vi "Test Device Under Test_Cloneable_DQMH API.vi"() -> ()   [LabVIEW 2015]
doc: "Device Under Test_Cloneable_DQMH API Tester.\n____\nDelacor QMH Thermal Chamber Examples 4.0.0.21\nCopyright (c) 2018, Delacor"
uses:
  Device Under Test_Cloneable_DQMH.lvlib
panel:
  in  "Run as Singleton?":bool
  out "timed out?":bool
  in  "Update DUT Status":bool
  out "Self Test Result":bool
  out "Power State":bool
  in  "Self Test":bool
  in  "Power Off":bool
  in  "Power On":bool
  in  "Show Block Diagram":bool
  in  "Refresh Modules":bool
  out "Active Modules":string[](array[string])
  in  "Stop Module":bool
  in  "Select Module":i32(ring)=-1 caption="Select Module\nTo send Request to" items=["All"=-1]
  in  "Run New Module":bool
  in  "Hide Module Panel":bool
  in  "Show Module Panel":bool
  out "Status":string
  # "This VI tests the API for the Module."
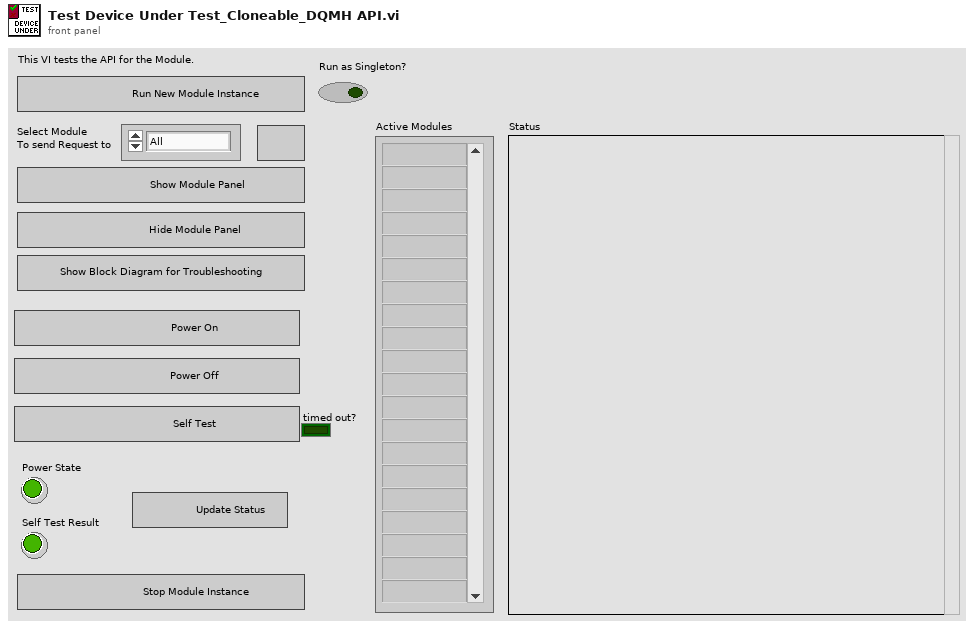
[diagram p1: front panel]
types:
  T1 = typedef "Device Under Test_Cloneable_DQMH.lvlib/Broadcast Events--cluster.ctl" = cluster{"Module Did Init":refnum<user-event>, "Status Updated":refnum<user-event>, "Error Reported":refnum<user-event>, "Module Did Stop":refnum<user-event>, "DUT Status Updated":refnum<user-event>, "Update Module Execution Status":refnum<user-event>}
  T2 = typedef "Device Under Test_Cloneable_DQMH.lvlib/Perform Self Test (Reply Payload)--cluster.ctl" = cluster{"Result":bool, "error":errorcluster}
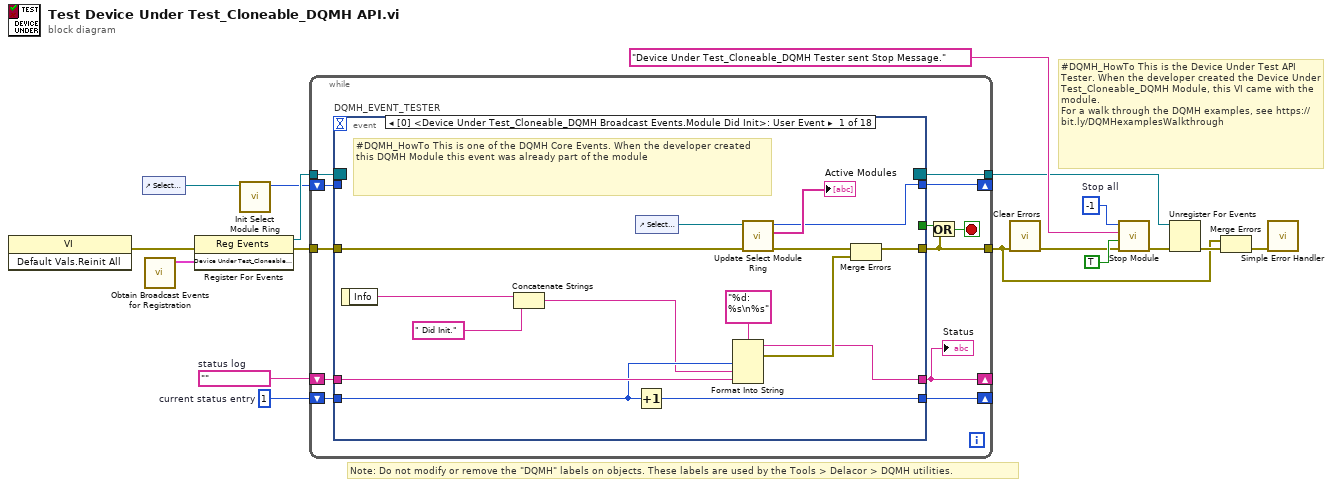
[diagram p0: block diagram]
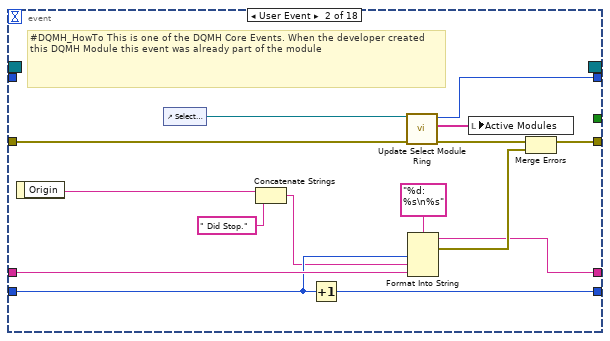
[diagram p2: hidden frame]
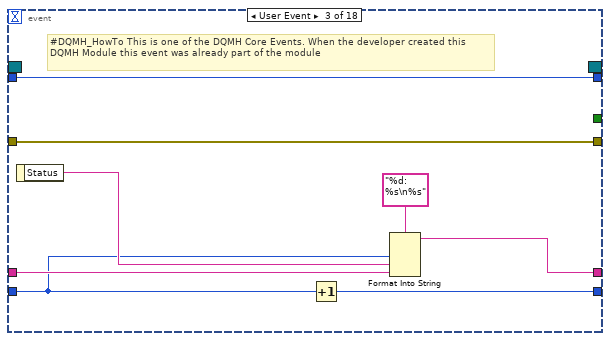
[diagram p3: hidden frame]
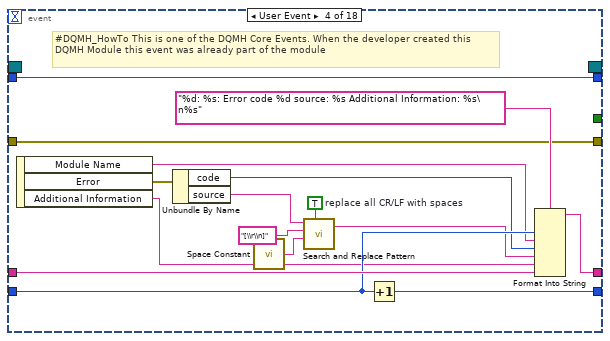
[diagram p4: hidden frame]
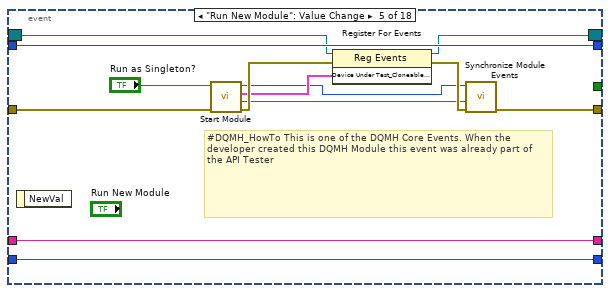
[diagram p5: hidden frame]
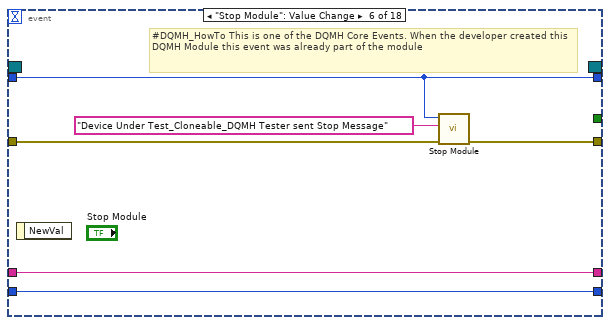
[diagram p6: hidden frame]
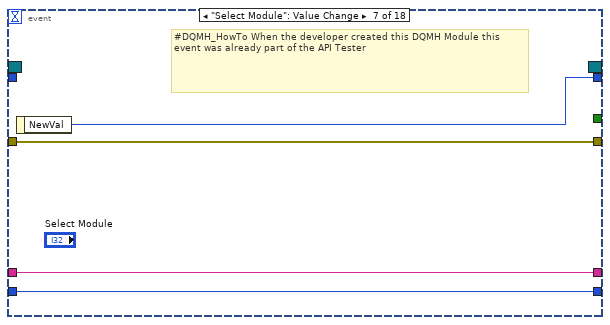
[diagram p7: hidden frame]
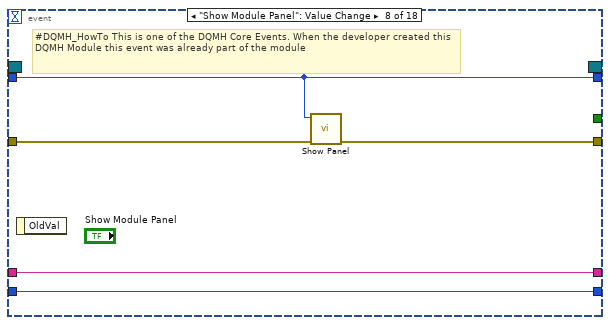
[diagram p8: hidden frame]
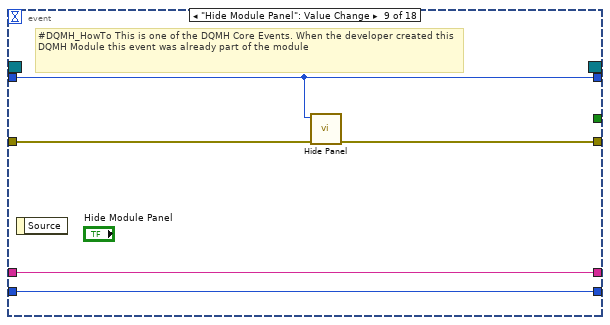
[diagram p9: hidden frame]
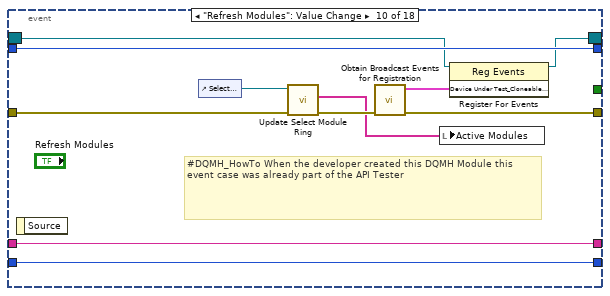
[diagram p10: hidden frame]
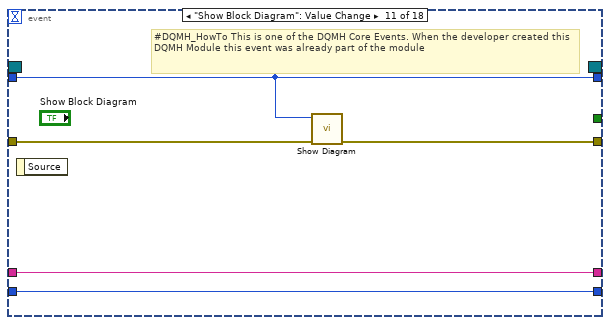
[diagram p11: hidden frame]
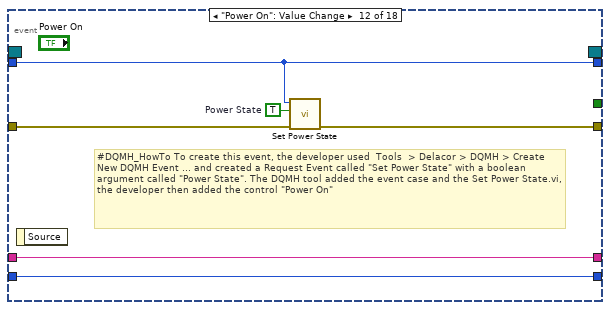
[diagram p12: hidden frame]
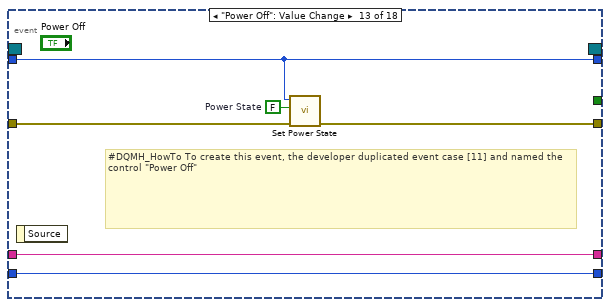
[diagram p13: hidden frame]
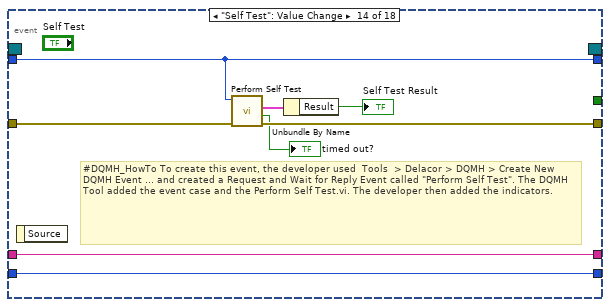
[diagram p14: hidden frame]
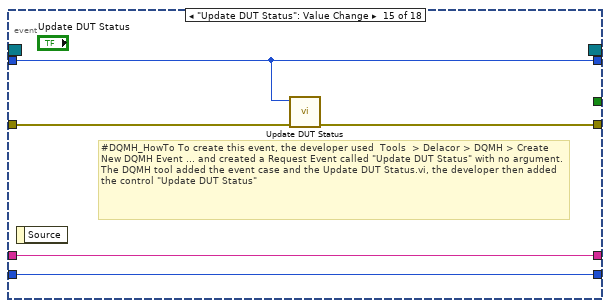
[diagram p15: hidden frame]
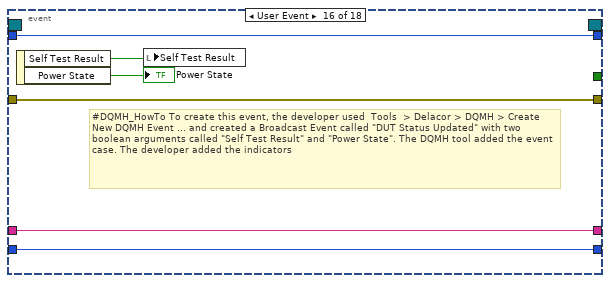
[diagram p16: hidden frame]
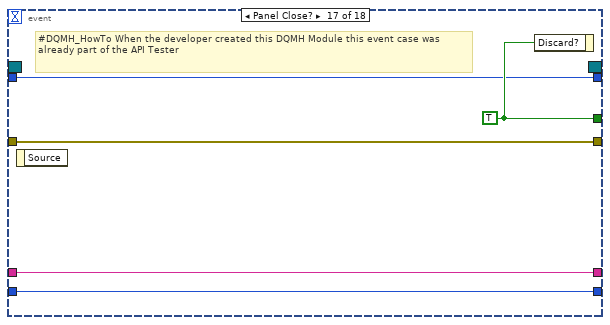
[diagram p17: hidden frame]
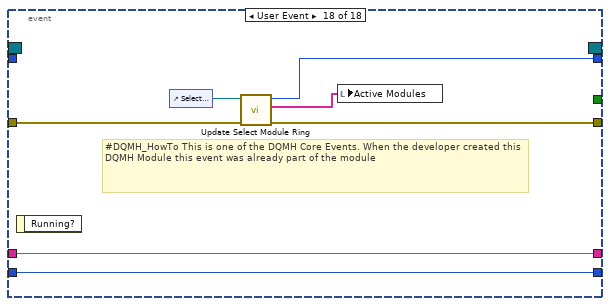
[diagram p18: hidden frame]
diagram:
  w7 = -1  # Stop all
  w13 = 1  # current status entry
  w14 = ""  # status log
  # "#DQMH_HowTo This is the Device Under Test API Tester. When the developer created the Device Under Test_Cloneable_DQMH Module, this VI came with the module.\nFor a walk through the DQMH examples, see https://bit.ly/DQMHexamplesWalkthrough"
  # "Note: Do not modify or remove the \"DQMH\" labels on objects. These labels are used by the Tools > Delacor > DQMH utilities."
  n1 = invoke class="VI" method="Default Vals.Reinit All"() -> (error out=w6:errorcluster)  [unwired: 3 in, 2 out]
  n2 = control-ref of="Select Module"() -> (w11:refnum<vi>)
  n3 = call "Obtain Broadcast Events for Registration.vi"() -> ("Device Under Test_Cloneable_DQMH Broadcast Events"=w10:T1)  [unwired: 10 in, 1 out]
  n4 = register-events(error in=w6, w10) -> (reference out=w17:refnum<event-registration>, error out=w9:errorcluster)  [unwired: 1 in]
  n5 = call "Init Select Module Ring.vi"("Select Module Ring Ref"=w11) -> ("Value for All Modules"=w12:i32)  [unwired: 8 in, 2 out]
  n6 = while {
    tunnel: w17 -> [w29]
    tunnel: [w19] -> w1
    tunnel: w9 -> [w27]
    shift-right: [w23] -> _
    shift-left: w14 -> [w25]
    shift-right: [w24] -> _
    shift-left: w13 -> [w26]
    shift-right: [w20] -> _
    shift-left: w12 -> [w21]
    tunnel: [w18] -> w5
    stop <- w22 stop-if-true
    n7 = event "DQMH_EVENT_TESTER" shown="[0] <Device Under Test_Cloneable_DQMH Broadcast Events.Module Did Init>: User Event" {
      selector: w29 -> [_ _ _ _ w90 _ _ _ _ w122 _ _ _ _ _ _ _ _]
      dyn-events: [_ _ _ _ w89 _ _ _ _ w121 _ _ _ _ _ _ _ _] -> w18
      timeout: _ -> [_ _ _ _ _ _ _ _ _ _ _ _ _ _ _ _ _ _]
      tunnel: [_ _ _ _ _ _ _ _ _ _ _ _ _ _ _ _ w168 _] -> w28
      tunnel: [w33 w51 w67 w73 w88 w98 w106 w110 w115 w118 w129 w135 w141 w149 w154 w163 w167 w172] -> w19
      tunnel: w27 -> [w35 w53 w67 w73 w91 w99 w106 w111 w116 w123 w132 w138 w144 w152 w157 w163 w167 w173]
      tunnel: w26 -> [w41 w56 w60 w79 w93 w101 w104 w108 w113 w126 w130 w136 w142 w150 w155 w161 w165 w174]
      tunnel: w25 -> [w42 w57 w63 w81 w94 w102 w105 w109 w114 w127 w131 w137 w143 w151 w156 w162 w166 w175]
      tunnel: [w39 w54 w64 w76 w94 w102 w105 w109 w114 w127 w131 w137 w143 w151 w156 w162 w166 w175] -> w23
      tunnel: [w40 w55 w66 w82 w93 w101 w104 w108 w113 w126 w130 w136 w142 w150 w155 w161 w165 w174] -> w24
      tunnel: w21 -> [_ _ w61 w83 w92 w100 _ w107 w112 w125 w128 w133 w139 w145 w153 w160 w164 _]
      tunnel: [w30 w48 w61 w83 w92 w100 w103 w107 w112 w125 w128 w133 w139 w145 w153 w160 w164 w170] -> w20
      event User Event {
        # "#DQMH_HowTo This is one of the DQMH Core Events. When the developer created this DQMH Module this event was already part of the module"
        n8 = event-data() -> ("Info"=w38:string)  [unwired: 1 in]
        n9 = Concatenate Strings(w38, " Did Init.") -> (w37:string)
        n10 = control-ref of="Select Module"() -> (w32:refnum<vi>)
        n11 = Increment(x=w41) -> (x+1=w40:i32)
        n12 = Format Into String(format string="%d: %s\n%s", w41, w37, w42) -> (resulting string=w39:string, error out=w44:errorcluster)  [unwired: 2 in]
        n13 = call "Update Select Module Ring.vi"("error in (no error)"=w35, "Select Module Ring Ref"=w32) -> ("error out"=w34:errorcluster, "Active Modules (Array)"=→"Active Modules":string[], "New Module Ring Value"=w30:i32)  [unwired: 7 in]
        n14 = Merge Errors(w34, w44) -> (w33:errorcluster)
      }
      event User Event {
        # "#DQMH_HowTo This is one of the DQMH Core Events. When the developer created this DQMH Module this event was already part of the module"
        n15 = event-data() -> ("Origin"=w46:string)  [unwired: 1 in]
        n16 = control-ref of="Select Module"() -> (w50:refnum<vi>)
        n17 = Concatenate Strings(w46, " Did Stop.") -> (w45:string)
        n18 = Increment(x=w56) -> (x+1=w55:i32)
        n19 = call "Update Select Module Ring.vi"("error in (no error)"=w53, "Select Module Ring Ref"=w50) -> ("error out"=w52:errorcluster, "Active Modules (Array)"=w49:string[], "New Module Ring Value"=w48:i32)  [unwired: 7 in]
        n20 = Format Into String(format string="%d: %s\n%s", w56, w45, w57) -> (resulting string=w54:string, error out=w59:errorcluster)  [unwired: 2 in]
        n21 = local write "Active Modules"(w49) -> ()
        n22 = Merge Errors(w52, w59) -> (w51:errorcluster)
      }
      event User Event {
        # "#DQMH_HowTo This is one of the DQMH Core Events. When the developer created this DQMH Module this event was already part of the module"
        n23 = event-data() -> ("Status"=w62:string)  [unwired: 1 in]
        n24 = Increment(x=w60) -> (x+1=w66:i32)
        n25 = Format Into String(format string="%d: %s\n%s", w60, w62, w63) -> (resulting string=w64:string)  [unwired: 2 in, 1 out]
      }
      event User Event {
        w77 = TRUE  # replace all CR/LF with spaces
        # "#DQMH_HowTo This is one of the DQMH Core Events. When the developer created this DQMH Module this event was already part of the module"
        n26 = event-data() -> ("Module Name"=w71:string, "Error"=w70:errorcluster, "Additional Information"=w68:string)  [unwired: 1 in]
        n27 = Unbundle By Name(w70) -> ("code"=w72:i32, "source"=w74:string)
        n28 = call <vilib>:"Space Constant.vi"() -> ("String"=w78:string)
        n29 = call <vilib>:"Search and Replace Pattern.vi"("string"=w74, "regular expression (\"\")"="[\\r\\n]" ("regular expression (\"\")"), "replace string (\"\")"=w78, "replace all? (F)"=w77) -> ("result string"=w75:string)  [unwired: 1 in, 1 out]
        n30 = Increment(x=w79) -> (x+1=w82:i32)
        n31 = Format Into String(format string="%d: %s: Error code %d source: %s Additional Information: %s\n%s", w79, w71, w72, w75, w68, w81) -> (resulting string=w76:string)  [unwired: 2 in, 1 out]
      }
      event "Run New Module": Value Change {
        # "#DQMH_HowTo This is one of the DQMH Core Events. When the developer created this DQMH Module this event was already part of the API Tester"
        n32 = event-data() -> ()  [unwired: 1 in, 1 out]
        n33 = call "Start Module.vi"("error in (no error)"=w91, "Run as Singleton? (F)"="Run as Singleton?") -> ("error out"=w95:errorcluster, "Wait for Event Sync?"=w87:bool, "Device Under Test_Cloneable_DQMH Broadcast Events"=w86:T1, "Module ID"=w84:i32)  [unwired: 6 in]
        n34 = register-events(reference=w90, error in=w95, w86) -> (reference out=w89:refnum<event-registration>, error out=w96:errorcluster)
        n35 = call "Synchronize Module Events.vi"("error in (no error)"=w96, "Wait for Event Sync?"=w87, "Module ID"=w84) -> ("error out"=w88:errorcluster)  [unwired: 7 in, 1 out]
      }
      event "Stop Module": Value Change {
        # "#DQMH_HowTo This is one of the DQMH Core Events. When the developer created this DQMH Module this event was already part of the module"
        n36 = event-data() -> ()  [unwired: 1 in, 1 out]
        n37 = call "Stop Module.vi"("error in (no error)"=w99, "Origin"="Device Under Test_Cloneable_DQMH Tester sent Stop Message", "Module ID"=w100) -> ("error out"=w98:errorcluster)  [unwired: 8 in]
      }
      event "Select Module": Value Change {
        # "#DQMH_HowTo When the developer created this DQMH Module this event was already part of the API Tester"
        n38 = event-data() -> ("NewVal"=w103:i32)  [unwired: 1 in]
      }
      event "Show Module Panel": Value Change {
        # "#DQMH_HowTo This is one of the DQMH Core Events. When the developer created this DQMH Module this event was already part of the module"
        n39 = event-data() -> ()  [unwired: 1 in, 1 out]
        n40 = call "Show Panel.vi"("error in (no error)"=w111, "Module ID"=w107) -> ("error out"=w110:errorcluster)  [unwired: 9 in]
      }
      event "Hide Module Panel": Value Change {
        # "#DQMH_HowTo This is one of the DQMH Core Events. When the developer created this DQMH Module this event was already part of the module"
        n41 = event-data() -> ()  [unwired: 1 in, 1 out]
        n42 = call "Hide Panel.vi"("error in (no error)"=w116, "Module ID"=w112) -> ("error out"=w115:errorcluster)  [unwired: 9 in]
      }
      event "Refresh Modules": Value Change {
        # "#DQMH_HowTo When the developer created this DQMH Module this event case was already part of the API Tester"
        n43 = event-data() -> ()  [unwired: 1 in, 1 out]
        n44 = control-ref of="Select Module"() -> (w124:refnum<vi>)
        n45 = call "Update Select Module Ring.vi"("error in (no error)"=w123, "Select Module Ring Ref"=w124) -> ("error out"=w119:errorcluster, "Active Modules (Array)"=w117:string[])  [unwired: 7 in, 1 out]
        n46 = call "Obtain Broadcast Events for Registration.vi"("error in (no error)"=w119) -> ("error out"=w118:errorcluster, "Device Under Test_Cloneable_DQMH Broadcast Events"=w120:T1)  [unwired: 9 in]
        n47 = local write "Active Modules"(w117) -> ()
        n48 = register-events(reference=w122, w120) -> (reference out=w121:refnum<event-registration>)  [unwired: 1 in, 1 out]
      }
      event "Show Block Diagram": Value Change {
        # "#DQMH_HowTo This is one of the DQMH Core Events. When the developer created this DQMH Module this event was already part of the module"
        n49 = event-data() -> ()  [unwired: 1 in, 1 out]
        n50 = call "Show Diagram.vi"("error in (no error)"=w132, "Module ID"=w128) -> ("error out"=w129:errorcluster)  [unwired: 9 in]
      }
      event "Power On": Value Change {
        w134 = TRUE  # Power State
        # "#DQMH_HowTo To create this event, the developer used  Tools  > Delacor > DQMH > Create New DQMH Event ... and created a Request Event called \"Set Power State\" with a boolean argument called \"Power State\". The DQMH tool added the event case and the Set Power State.vi, the developer then added the control \"Power On\""
        n51 = event-data() -> ()  [unwired: 1 in, 1 out]
        n52 = call "Set Power State.vi"("error in (no error)"=w138, "Power State"=w134, "Module ID"=w133) -> ("error out"=w135:errorcluster)  [unwired: 8 in]
      }
      event "Power Off": Value Change {
        w140 = FALSE  # Power State
        # "#DQMH_HowTo To create this event, the developer duplicated event case [11] and named the control \"Power Off\""
        n53 = event-data() -> ()  [unwired: 1 in, 1 out]
        n54 = call "Set Power State.vi"("error in (no error)"=w144, "Power State"=w140, "Module ID"=w139) -> ("error out"=w141:errorcluster)  [unwired: 8 in]
      }
      event "Self Test": Value Change {
        # "#DQMH_HowTo To create this event, the developer used  Tools  > Delacor > DQMH > Create New DQMH Event ... and created a Request and Wait for Reply Event called \"Perform Self Test\". The DQMH Tool added the event case and the Perform Self Test.vi. The developer then added the indicators."
        n55 = event-data() -> ()  [unwired: 1 in, 1 out]
        n56 = call "Perform Self Test.vi"("error in (no error)"=w152, "Module ID"=w145) -> ("error out"=w149:errorcluster, "timed out?"=→"timed out?":bool, "Reply Payload"=w148:T2)  [unwired: 7 in]
        n57 = Unbundle By Name(w148) -> ("Result"=→"Self Test Result":bool)
      }
      event "Update DUT Status": Value Change {
        # "#DQMH_HowTo To create this event, the developer used  Tools  > Delacor > DQMH > Create New DQMH Event ... and created a Request Event called \"Update DUT Status\" with no argument. The DQMH tool added the event case and the Update DUT Status.vi, the developer then added the control \"Update DUT Status\""
        n58 = event-data() -> ()  [unwired: 1 in, 1 out]
        n59 = call "Update DUT Status.vi"("error in (no error)"=w157, "Module ID"=w153) -> ("error out"=w154:errorcluster)  [unwired: 9 in]
      }
      event User Event {
        # "#DQMH_HowTo To create this event, the developer used  Tools  > Delacor > DQMH > Create New DQMH Event ... and created a Broadcast Event called \"DUT Status Updated\" with two boolean arguments called \"Self Test Result\" and \"Power State\". The DQMH tool added the event case. The developer added the indicators"
        n60 = event-data() -> ("Self Test Result"=w158:bool, "Power State"=→"Power State":bool)  [unwired: 1 in]
        n61 = local write "Self Test Result"(w158) -> ()
      }
      event Panel Close? {
        w168 = TRUE ("Discard?")
        # "#DQMH_HowTo When the developer created this DQMH Module this event case was already part of the API Tester"
        n62 = event-data() -> ()  [unwired: 1 in, 1 out]
        n63 = event-data("Discard?"=w168) -> ()  [unwired: 1 in, 1 out]
      }
      event User Event {
        # "#DQMH_HowTo This is one of the DQMH Core Events. When the developer created this DQMH Module this event was already part of the module"
        n64 = event-data() -> ()  [unwired: 1 in, 1 out]
        n65 = control-ref of="Select Module"() -> (w169:refnum<vi>)
        n66 = call "Update Select Module Ring.vi"("error in (no error)"=w173, "Select Module Ring Ref"=w169) -> ("error out"=w172:errorcluster, "Active Modules (Array)"=w171:string[], "New Module Ring Value"=w170:i32)  [unwired: 7 in]
        n67 = local write "Active Modules"(w171) -> ()
      }
    }
    "Status" <- w23
    n68 = Or(x=w28, y=w19) -> (x .or. y?=w22:bool)
  }
  n69 = call <vilib>:"Clear Errors.vi"("error in (no error)"=w1) -> ("error out"=w3:errorcluster)  [unwired: 5 in, 1 out]
  n70 = call "Stop Module.vi"("error in (no error)"=w3, "Wait for Module to stop? (F)"=TRUE ("Wait for Module to stop?"), "Origin"="Device Under Test_Cloneable_DQMH Tester sent Stop Message.", "Module ID"=w7) -> ("error out"=w15:errorcluster)  [unwired: 7 in]
  n71 = Unregister For Events(event registration refnum=w5, error in=w15) -> (error out=w16:errorcluster)
  n72 = Merge Errors(w1, w16) -> (w2:errorcluster)
  n73 = call <vilib>:"Simple Error Handler.vi"("error in (no error)"=w2) -> ()  [unwired: 4 in, 5 out]
